vi "FTW-TransferClient-Callback-StatusDownload.vi"(4 "Initial Parameters":T1 {"Initial Time" format="%.4psec"}, 5 "Event Data":cluster{"sender":refnum<k24>, "e":refnum<k24>}, 6 "Control Ref":refnum<k24>, 7 "Event Common Data":T2) -> ()   [LabVIEW 2015]
uses:
  FTW-TransferClient-TransferStatus.ctl
panel:
  # "Inputs"
  # "Outputs"
  # "No Outputs - this VI\nis fire and forget"
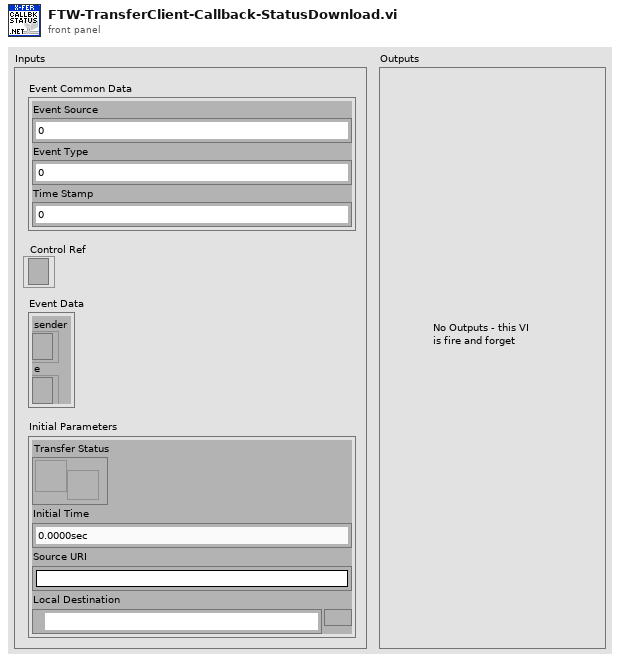
[diagram p1: front panel]
types:
  T1 = cluster{"Transfer Status":refnum<user-event>, "Initial Time":dbl, "Source URI":string, "Local Destination":path}
  T2 = cluster{"Event Source":i32, "Event Type":u32, "Time Stamp":u32}
  T3 = typedef "FTW-TransferClient-TransferStatus.ctl" = cluster{"Remote URI":string, "Local Filepath":path, "Cancelled?":bool, "Error?":bool, "Error Message":string, "Elapsed Time":dbl}
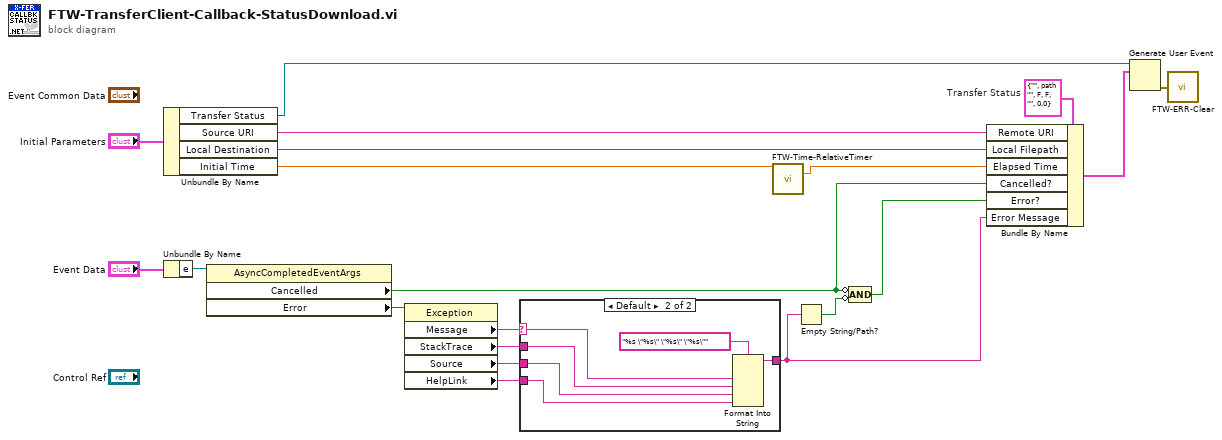
[diagram p0: block diagram]
diagram:
  w10 = T3 {"Remote URI"="", "Local Filepath"=path "", "Cancelled?"=FALSE, "Error?"=FALSE, "Error Message"="", "Elapsed Time"=0.0}  # Transfer Status
  n1 = Unbundle By Name("Initial Parameters") -> ("Transfer Status"=w4:refnum<user-event>, "Source URI"=w3:string, "Local Destination"=w2:path, "Initial Time"=w1:dbl)
  n2 = Unbundle By Name("Event Data") -> ("e"=w18:refnum<k24>)
  n3 = property class="AsyncCompletedEventArgs"(reference=w18) -> ("Cancelled"=w5:bool, "Error"=w6:refnum<k24>)  [unwired: 1 in, 2 out]
  n4 = property class="Exception"(reference=w6) -> ("Message"=w15:string, "StackTrace"=w16:string, "Source"=w14:string, "HelpLink"=w13:string)  [unwired: 1 in, 2 out]
  n5 = case shown="Default" w15 {
    selector: w15 -> [_ w24]
    tunnel: w16 -> [_ w23]
    tunnel: [_ w25] -> w8
    tunnel: w14 -> [_ w22]
    tunnel: w13 -> [_ w21]
    frame "" {
    }
    frame Default {
      n6 = Format Into String(format string="%s \"%s\" \"%s\" \"%s\"", w24, w23, w22, w21) -> (resulting string=w25:string)  [unwired: 2 in, 1 out]
    }
  }
  n7 = call "FTW-Time-RelativeTimer.vi"("Previous Timer Value"=w1) -> ("Elapsed Time"=w7:dbl)  [unwired: 12 in, 2 out]
  n8 = Empty String/Path?(string/path=w8) -> (empty?=w17:bool)
  n9 = Compound Arithmetic op=AND(invert w5, invert w17) -> (w9:bool)
  n10 = Bundle By Name(cluster=w10, "Remote URI"=w3, "Local Filepath"=w2, "Elapsed Time"=w7, "Cancelled?"=w5, "Error?"=w9, "Error Message"=w8) -> (w12:T3)
  n11 = Generate User Event(user event=w4, event data cluster=w12) -> (error out=w11:errorcluster)  [unwired: 2 in, 1 out]
  n12 = call "FTW-ERR-Clear.vi"("error to snuff"=w11) -> ()  [unwired: 1 out]
